vi "reconfigure.vi"() -> ()   [LabVIEW 2011]
panel:
  out "Function List":T1(array[cluster])
  out "error out":errorcluster
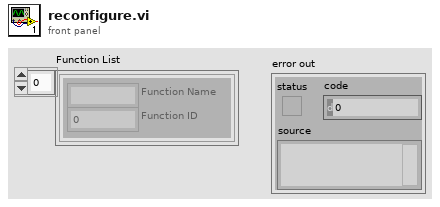
[diagram p1: front panel]
types:
  T1 = cluster{"Function Name":string, "Function ID":u32}[]
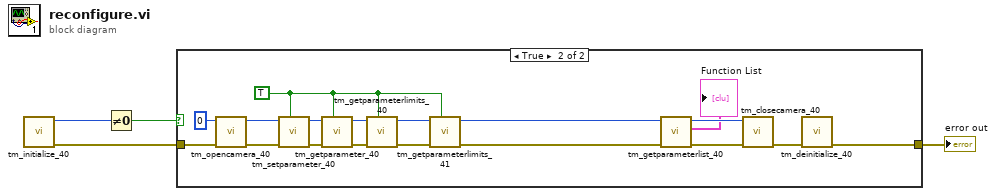
[diagram p0: block diagram]
diagram:
  n1 = call <userlib>:"tm_initialize_40.vi"() -> ("error out"=w3:errorcluster, "Number Of Cameras"=w4:u32)  [unwired: 8 in, 2 out]
  n2 = Not Equal To 0?(x=w4) -> (x != 0?=w2:bool)
  n3 = case shown="True" w2 {
    tunnel: w3 -> [w5 w23]
    tunnel: [w5 w14] -> w1
    frame False {
    }
    frame True {
      w6 = TRUE ("Reconfigure (F)")
      n4 = call <userlib>:"tm_opencamera_40.vi"("error in (no error)"=w23, "Camera Index"=u32 0) -> ("error out"=w21:errorcluster, "Handle out"=w20:u32)  [unwired: 7 in, 1 out]
      n5 = call <userlib>:"tm_setparameter_40.vi"("Reconfigure (F)"=w6, "error in (no error)"=w21, "Handle in"=w20) -> ("error out"=w19:errorcluster, "Handle out"=w18:u32)  [unwired: 7 in]
      n6 = call <userlib>:"tm_getparameter_40.vi"("Reconfigure (F)"=w6, "error in (no error)"=w19, "Handle in"=w18) -> ("error out"=w16:errorcluster, "Handle out"=w17:u32)  [unwired: 6 in, 1 out]
      n7 = call <userlib>:"tm_getparameterlimits_40.vi"("Reconfigure (F)"=w6, "error in (no error)"=w16, "Handle in"=w17) -> ("error out"=w10:errorcluster, "Handle out"=w9:u32)  [unwired: 2 in, 5 out]
      n8 = call <userlib>:"tm_getparameterlimits_41.vi"("Reconfigure (F)"=w6, "error in (no error)"=w10, "Handle in"=w9) -> ("error out"=w7:errorcluster, "Handle out"=w8:u32)  [unwired: 6 in, 1 out]
      n9 = call <userlib>:"tm_getparameterlist_40.vi"("error in (no error)"=w7, "Handle in"=w8) -> ("error out"=w12:errorcluster, "Function List"=→"Function List":T1, "Handle out"=w13:u32)  [unwired: 7 in]
      n10 = call <userlib>:"tm_closecamera_40.vi"("error in (no error)"=w12, "Handle in"=w13) -> ("error out"=w15:errorcluster)  [unwired: 9 in]
      n11 = call <userlib>:"tm_deinitialize_40.vi"("error in (no error)"=w15) -> ("error out"=w14:errorcluster)  [unwired: 10 in]
    }
  }
  "error out" <- w1
